vi "_main_factoryMethod.vi"() -> ()   [LabVIEW 2023]
uses:
  LegacyOvenController/LegacyOvenController.lvclass
  ModernOvenController/ModernOvenController.lvclass
  OvenController/OvenController.lvclass
panel:
  in  "newTemperature(TCP)":dbl=123.0
  in  "newTemperature(serial)":dbl=85.0
  # "FACTORY METHOD"
  # "INSTRUCTIONS:\n- Set the desired temperature for both the Legacy and the Moder oven.\n- Run the code.\n- See comments in the block diagram"
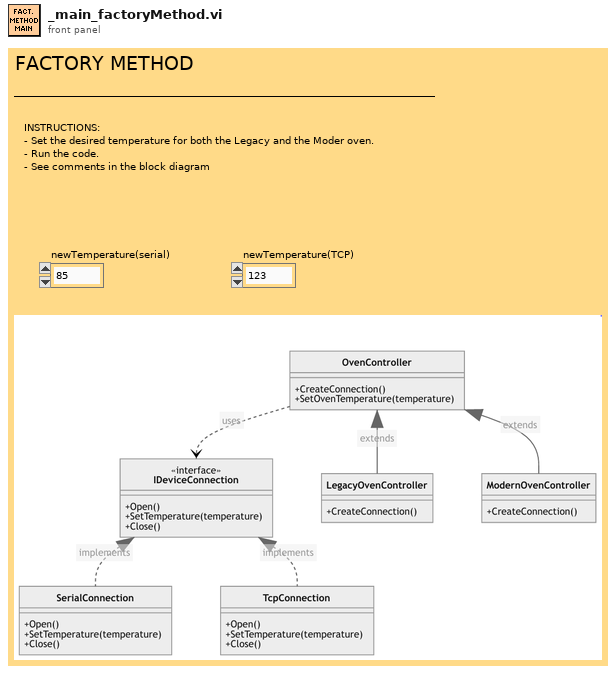
[diagram p1: front panel]
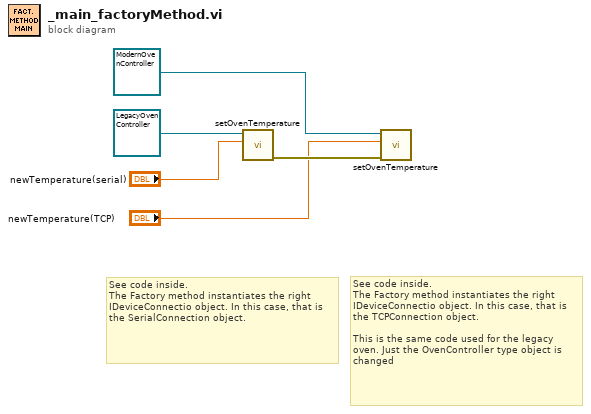
[diagram p0: block diagram]
diagram:
  # "See code inside. \nThe Factory method instantiates the right IDeviceConnectio object. In this case, that is the TCPConnection object.\n\nThis is the same code used for the legacy oven. Just the OvenController type object is changed"
  # "See code inside. \nThe Factory method instantiates the right IDeviceConnectio object. In this case, that is the SerialConnection object."
  n1 = call "setOvenTemperature.vi"("temperature"="newTemperature(serial)", "OvenController in"=refnum<class "LegacyOvenController.lvclass"> refnum ("LegacyOvenController.lvclass")) -> ("error out"=w3:errorcluster)  [unwired: 8 in, 1 out]
  n2 = call "setOvenTemperature.vi"("error in (no error)"=w3, "temperature"="newTemperature(TCP)", "OvenController in"=refnum<class "ModernOvenController.lvclass"> refnum ("ModernOvenController.lvclass")) -> ()  [unwired: 7 in, 2 out]
